vi "Event Based Read.vi"() -> ()   [LabVIEW 2020]
uses:
  <vilib>/DAQmx/read.llb/DAQmx Read (Analog Wfm 1Chan NSamp).vi
  <vilib>/DAQmx/create/channels.llb/DAQmx Create Channel (AI-Voltage-Basic).vi
  <vilib>/DAQmx/configure/timing.llb/DAQmx Timing (Sample Clock).vi
  <vilib>/DAQmx/miscellaneous.llb/DAQmx Fill In Error Info.vi
panel:
  in  "Loop Rate (<100)":u32=1
  out "Time In Read":dbl(graph)
  in  "stop":bool
  in  "Event Based":bool
  in  "Sample Rate":u32=100
  out "error out":errorcluster
  out "Waveform":waveform(dbl)(graph)
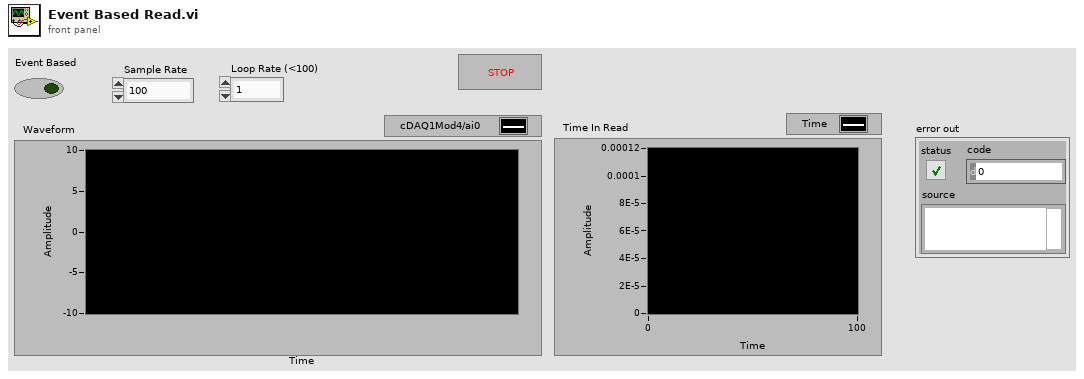
[diagram p1: front panel]
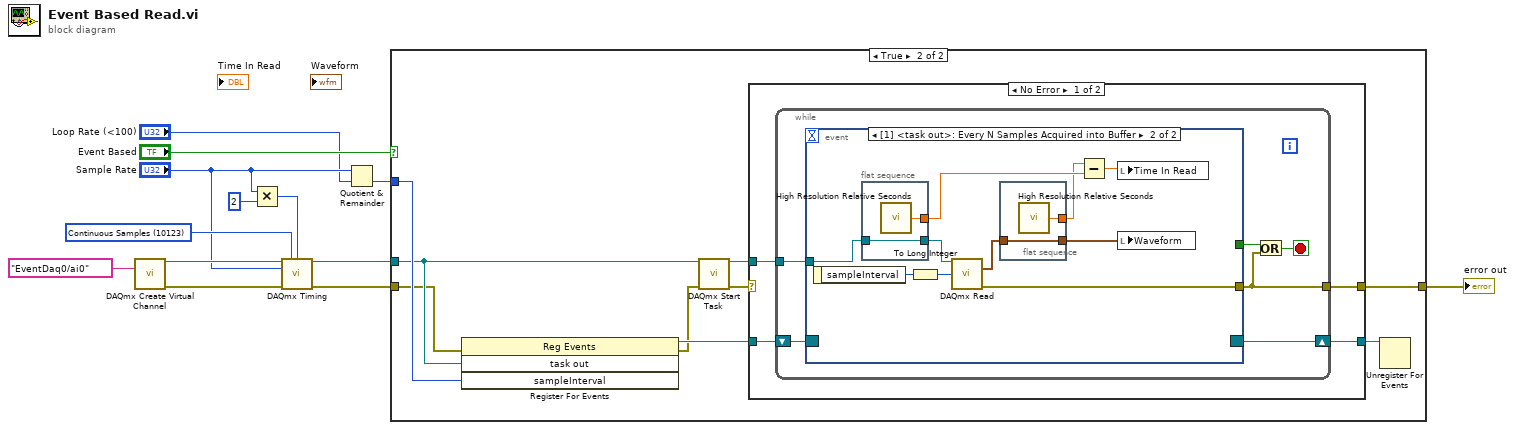
[diagram p0: block diagram]
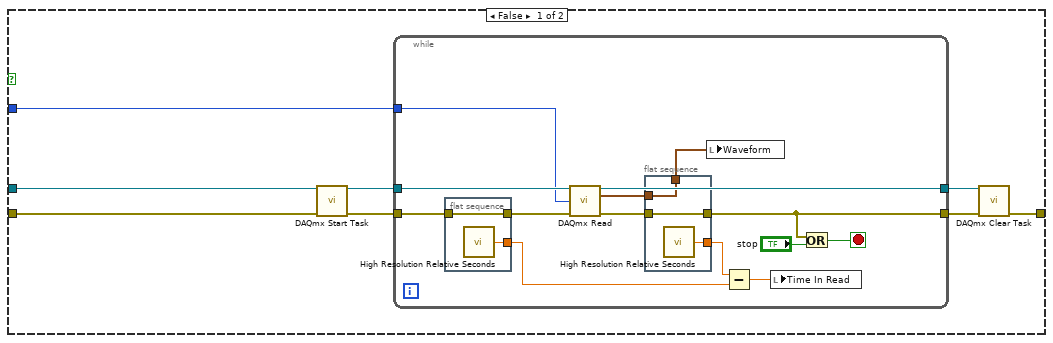
[diagram p2: hidden frame]
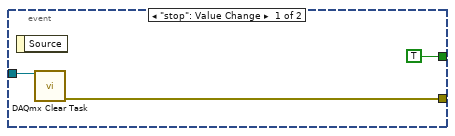
[diagram p3: hidden frame]
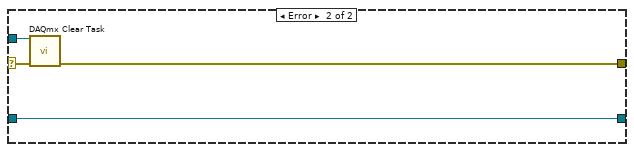
[diagram p4: hidden frame]
diagram:
  w7 = 10123 items=["Finite Samples"=10178, "Continuous Samples"=10123, "Hardware Timed Single Point"=12522] ("sample mode")
  n1 = call-poly <vilib>:"DAQmx Create Virtual Channel.vi"("physical channels"=tag "EventDaq0/ai0") -> ("task out"=w12:refnum<k21>, "error out"=w11:errorcluster)  [unwired: 13 in]
  n2 = Multiply(x="Sample Rate", y=u32 2) -> (x*y=w3:u32)
  n3 = call-poly <vilib>:"DAQmx Timing.vi"("task/channels in"=w12, "sample mode"=w7, "samples per channel"=w3, "rate"="Sample Rate", "error in"=w11) -> ("task out"=w9:refnum<k21>, "error out"=w10:errorcluster)  [unwired: 9 in]
  n4 = Quotient & Remainder(x="Sample Rate", y="Loop Rate (<100)") -> (floor(x/y)=w2:u32)  [unwired: 1 out]
  n5 = case shown="True" "Event Based" {
    tunnel: w10 -> [w20 w41]
    tunnel: w9 -> [w21 w42]
    tunnel: [w14 w45] -> w8
    tunnel: w2 -> [w17 w43]
    frame False {
      n6 = call <vilib>:"DAQmx Start Task.vi"("task/channels in"=w21, "error in"=w20) -> ("task out"=w19:refnum<k21>, "error out"=w18:errorcluster)  [unwired: 12 in]
      n7 = while {
        tunnel: w17 -> [w32]
        tunnel: w19 -> [w33]
        tunnel: [w31] -> w16
        tunnel: w18 -> [w30]
        tunnel: [w26] -> w15
        stop <- w34 stop-if-true
        n8 = flat-sequence {
          tunnel: w30 -> [w40]
          tunnel: [w40] -> w29
          tunnel: [w39] -> w23
          frame #0 {
            n9 = call <vilib>:"High Resolution Relative Seconds.vi"() -> ("relative seconds"=w39:dbl)
          }
        }
        n10 = call-poly <vilib>:"DAQmx Read.vi"("task/channels in"=w33, "number of samples per channel"=w32, "error in"=w29) -> ("task out"=w31:refnum<k21>, "data"=w27:waveform(dbl), "error out"=w28:errorcluster)  [unwired: 10 in]
        n11 = flat-sequence {
          tunnel: w28 -> [w38]
          tunnel: [w38] -> w26
          tunnel: w27 -> [w37]
          tunnel: [w37] -> w25
          tunnel: [w36] -> w24
          frame #0 {
            n12 = call <vilib>:"High Resolution Relative Seconds.vi"() -> ("relative seconds"=w36:dbl)
          }
        }
        n13 = local write "Waveform"(w25) -> ()
        n14 = Subtract(x=w24, y=w23) -> (x-y=w22:dbl)
        n15 = local write "Time In Read"(w22) -> ()
        n16 = Or(x=w26, y="stop") -> (x .or. y?=w34:bool)
      }
      n17 = call <vilib>:"DAQmx Clear Task.vi"("task in"=w16, "error in"=w15) -> ("error out"=w14:errorcluster)  [unwired: 13 in]
    }
    frame True {
      n18 = register-events(error in=w41, w42, w43) -> (reference out=w49:refnum<event-registration>, error out=w48:errorcluster)  [unwired: 1 in]
      n19 = call <vilib>:"DAQmx Start Task.vi"("task/channels in"=w42, "error in"=w48) -> ("task out"=w47:refnum<k21>, "error out"=w46:errorcluster)  [unwired: 12 in]
      n20 = case shown="No Error" w46 {
        selector: w46 -> [_ w78]
        tunnel: w49 -> [w53 w80]
        tunnel: w47 -> [w52 w79]
        tunnel: [w51 w80] -> w44
        tunnel: [w50 w77] -> w45
        frame No Error {
          n21 = while {
            tunnel: w52 -> [w58]
            shift-right: [w57] -> w51
            shift-left: w53 -> [w59]
            tunnel: [w54] -> w50
            stop <- w55 stop-if-true
            n22 = event shown="[1] <task out>: Every N Samples Acquired into Buffer" {
              selector: w59 -> [_ _]
              dyn-events: [_ _] -> w57
              timeout: _ -> [_ _]
              tunnel: w58 -> [w61 w69]
              tunnel: [TRUE ("Discard?") _] -> w56
              tunnel: [w60 w70] -> w54
              event "stop": Value Change {
                n23 = event-data() -> ()  [unwired: 1 in, 1 out]
                n24 = call <vilib>:"DAQmx Clear Task.vi"("task in"=w61) -> ("error out"=w60:errorcluster)  [unwired: 14 in]
              }
              event Every N Samples Acquired into Buffer {
                n25 = event-data() -> ("sampleInterval"=w72:u32)  [unwired: 1 in]
                n26 = flat-sequence {
                  tunnel: [w76] -> w65
                  tunnel: w69 -> [w75]
                  tunnel: [w75] -> w68
                  frame #0 {
                    n27 = call <vilib>:"High Resolution Relative Seconds.vi"() -> ("relative seconds"=w76:dbl)
                  }
                }
                n28 = To Long Integer(number=w72) -> (32bit integer=w71:i32)
                n29 = call-poly <vilib>:"DAQmx Read.vi"("task/channels in"=w68, "number of samples per channel"=w71) -> ("data"=w67:waveform(dbl), "error out"=w70:errorcluster)  [unwired: 11 in, 1 out]
                n30 = flat-sequence {
                  tunnel: [w74] -> w64
                  tunnel: w67 -> [w73]
                  tunnel: [w73] -> w66
                  frame #0 {
                    n31 = call <vilib>:"High Resolution Relative Seconds.vi"() -> ("relative seconds"=w74:dbl)
                  }
                }
                n32 = Subtract(x=w64, y=w65) -> (x-y=w63:dbl)
                n33 = local write "Time In Read"(w63) -> ()
                n34 = local write "Waveform"(w66) -> ()
              }
            }
            n35 = Or(x=w56, y=w54) -> (x .or. y?=w55:bool)
          }
        }
        frame Error {
          n36 = call <vilib>:"DAQmx Clear Task.vi"("task in"=w79, "error in"=w78) -> ("error out"=w77:errorcluster)  [unwired: 13 in]
        }
      }
      n37 = Unregister For Events(event registration refnum=w44) -> ()  [unwired: 1 in, 1 out]
    }
  }
  "error out" <- w8
